vi "SearchFolders.vi"(8 "error in":errorcluster, 9 "Folder":string="TrainData", 10 "regular expression":string="SwtX", 11 "file path":path=path "D:/Minecraft/mmc-stable-win32/MultiMC/instances/TRAINS 3-/.minecraft/saves/trains/opencomputers/442cd0d6-e139-46e7-881b-600456d36bc7/home") -> (0 "error out":errorcluster, 2 "File Array":string[](array[string]), 3 "Path Array":path[](array[path]), 5 "Root Path Array":path[](array[path]))   [LabVIEW 2014]
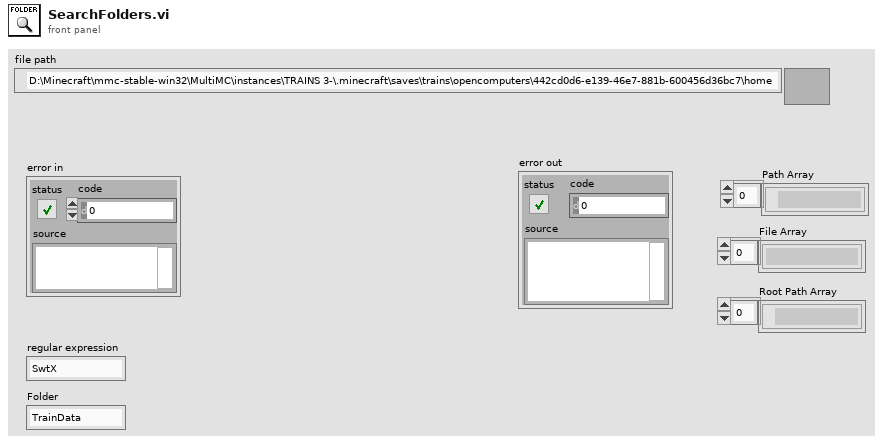
[diagram p1: front panel]
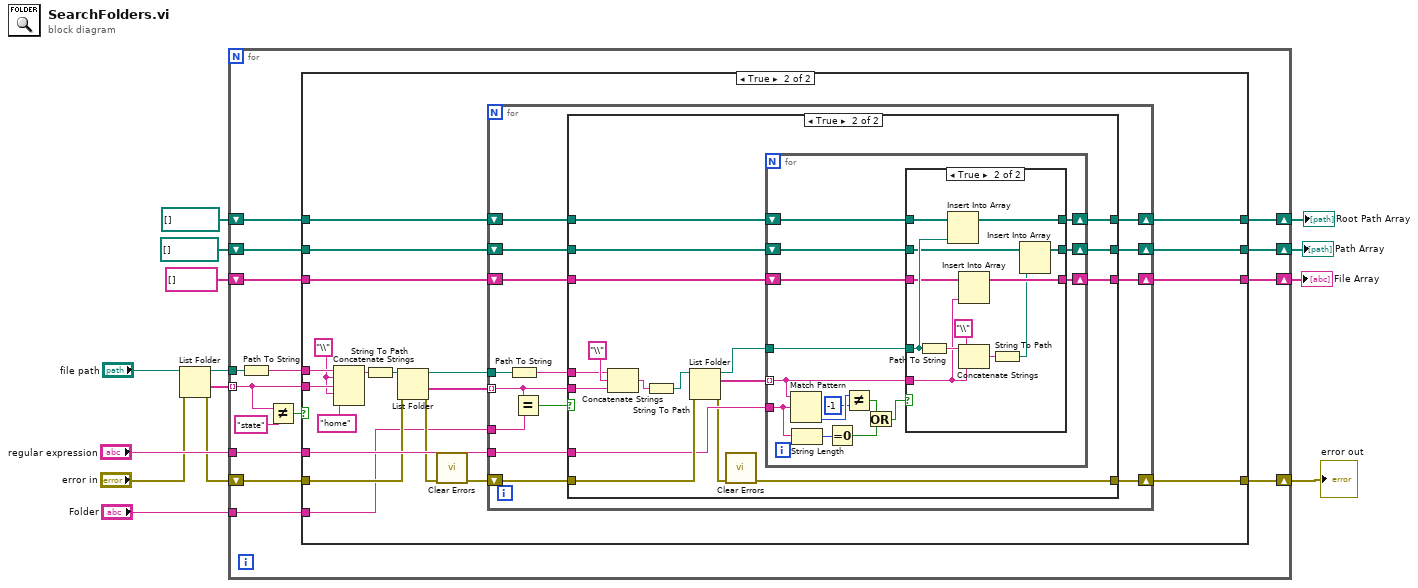
[diagram p0: block diagram]
diagram:
  n1 = List Folder(path="file path", error in="error in") -> (path out=w7:path, folder names=w8:string[], error out=w6:errorcluster)  [unwired: 2 in, 1 out]
  n2 = for {
    tunnel: w8 -> [w27] mode=indexing
    tunnel: w7 -> [w26]
    tunnel: "regular expression" -> [w24]
    shift-right: [w23] -> w12
    shift-left: w6 -> [w22]
    shift-right: [w21] -> w5
    shift-left: path[] [] -> [w20]
    shift-right: [w19] -> w9
    shift-left: path[] [] -> [w18]
    shift-right: [w17] -> w10
    shift-left: string[] [] -> [w16]
    tunnel: "Folder" -> [w15]
    n3 = Path To String(path=w26) -> (string=w25:string)
    n4 = Not Equal?(x=w27, y="state") -> (x != y?=w28:bool)
    n5 = case shown="True" w28 {
      tunnel: w27 -> [_ w52]
      tunnel: w25 -> [_ w53]
      tunnel: w22 -> [w33 w37]
      tunnel: w24 -> [_ w50]
      tunnel: [w33 w47] -> w23
      tunnel: [w32 w46] -> w21
      tunnel: w20 -> [w32 w43]
      tunnel: [w31 w45] -> w19
      tunnel: w18 -> [w31 w41]
      tunnel: [w30 w44] -> w17
      tunnel: w16 -> [w30 w42]
      tunnel: w15 -> [_ w34]
      frame False {
      }
      frame True {
        w49 = "\\" ("string")
        n6 = Concatenate Strings(w53, w49, w52, w49, "home" ("string")) -> (w51:string)
        n7 = String To Path(string=w51) -> (path=w40:path)
        n8 = List Folder(path=w40, error in=w37) -> (path out=w38:path, folder names=w39:string[], error out=w36:errorcluster)  [unwired: 2 in, 1 out]
        n9 = call <vilib>:"Clear Errors.vi"("error in (no error)"=w36) -> ("error out"=w35:errorcluster)  [unwired: 5 in, 1 out]
        n10 = for {
          tunnel: w50 -> [w66]
          shift-right: [w65] -> w47
          shift-left: w35 -> [w67]
          tunnel: w39 -> [w57] mode=indexing
          tunnel: w38 -> [w56]
          shift-right: [w62] -> w44
          shift-left: w42 -> [w60]
          shift-right: [w63] -> w45
          shift-left: w41 -> [w59]
          shift-right: [w64] -> w46
          shift-left: w43 -> [w61]
          tunnel: w34 -> [w54]
          n11 = Path To String(path=w56) -> (string=w55:string)
          n12 = Equal?(x=w57, y=w54) -> (x = y?=w58:bool)
          n13 = case shown="True" w58 {
            tunnel: w67 -> [w68 w87]
            tunnel: w66 -> [_ w86]
            tunnel: [w68 w84] -> w65
            tunnel: [w71 w83] -> w64
            tunnel: [w70 w82] -> w63
            tunnel: [w69 w81] -> w62
            tunnel: w61 -> [w71 w80]
            tunnel: w60 -> [w69 w79]
            tunnel: w59 -> [w70 w78]
            tunnel: w57 -> [_ w76]
            tunnel: w55 -> [_ w75]
            frame False {
            }
            frame True {
              n14 = Concatenate Strings(w75, "\\" ("string"), w76) -> (w74:string)
              n15 = String To Path(string=w74) -> (path=w73:path)
              n16 = List Folder(path=w73, error in=w87) -> (path out=w88:path, filenames=w72:string[], error out=w85:errorcluster)  [unwired: 2 in, 1 out]
              n17 = call <vilib>:"Clear Errors.vi"("error in (no error)"=w85) -> ("error out"=w84:errorcluster)  [unwired: 5 in, 1 out]
              n18 = for {
                tunnel: w72 -> [w99] mode=indexing
                tunnel: w88 -> [w103]
                tunnel: w86 -> [w93]
                shift-right: [w97] -> w83
                shift-left: w80 -> [w96]
                shift-right: [w102] -> w82
                shift-left: w78 -> [w95]
                shift-right: [w98] -> w81
                shift-left: w79 -> [w94]
                n19 = Match Pattern(string=w99, regular expression=w93) -> (offset past match=w101:i32)  [unwired: 1 in, 3 out]
                n20 = String Length(string=w93) -> (length=w92:i32)
                n21 = Equal To 0?(x=w92) -> (x = 0?=w91:bool)
                n22 = Not Equal?(x=w101, y=-1) -> (x != y?=w90:bool)
                n23 = Or(x=w90, y=w91) -> (x .or. y?=w89:bool)
                n24 = case shown="True" w89 {
                  tunnel: w103 -> [_ w114]
                  tunnel: [w105 w107] -> w102
                  tunnel: w99 -> [_ w111]
                  tunnel: [w104 w110] -> w98
                  tunnel: [w106 w113] -> w97
                  tunnel: w96 -> [w106 w115]
                  tunnel: w95 -> [w105 w109]
                  tunnel: w94 -> [w104 w112]
                  frame False {
                  }
                  frame True {
                    n25 = Path To String(path=w114) -> (string=w117:string)
                    n26 = Insert Into Array(array=w115, new element=w114) -> (w113:path[])  [unwired: 1 in]
                    n27 = Insert Into Array(array=w112, new element=w111) -> (w110:string[])  [unwired: 1 in]
                    n28 = Concatenate Strings(w117, "\\" ("string"), w111) -> (w116:string)
                    n29 = String To Path(string=w116) -> (path=w108:path)
                    n30 = Insert Into Array(array=w109, new element=w108) -> (w107:path[])  [unwired: 1 in]
                  }
                }
              }
            }
          }
        }
      }
    }
  }
  "error out" <- w12
  "File Array" <- w10
  "Path Array" <- w9
  "Root Path Array" <- w5
